vi "String_Subset.vi"() -> ()   [LabVIEW 2019]
panel:
  out "Result":string
  in  "String":string="Ankit Dudharejiya"
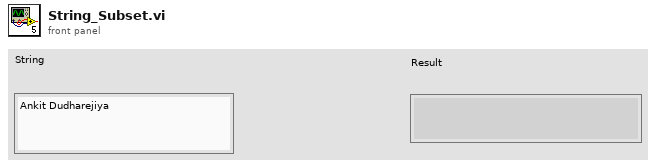
[diagram p1: front panel]
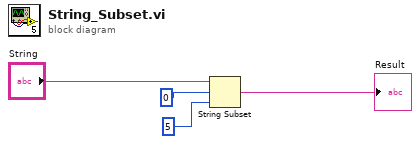
[diagram p0: block diagram]
diagram:
  n1 = String Subset(string="String", offset (0)=0, length (rest)=5 ("length (rest)")) -> (substring=→"Result":string)
